vi "Initialize.vi"(7 "Serial Configuration":T1={"Baud Rate"=9600, "Parity"=1, "Data Bits"=7, "Stop Bits"=10, "Flow Control"=0} {"Flow Control" items=["None", "XON/XOFF", "RTS/CTS", "XON/XOFF & RTS/CTS", "DTR/DSR", "XON/XOFF & DTR/DSR"]; "Stop Bits" items=["1.0"=10, "1.5"=15, "2.0"=20]; "Data Bits" items=["7"=7, "8"=8]; "Parity" items=["None", "Odd", "Even", "Mark", "Space"]; "Baud Rate" items=["300"=300, "600"=600, "1200"=1200, "2400"=2400, "4800"=4800, "9600"=9600, "19200"=19200, "38400"=38400, "57600"=57600]}, 8 "error in (no error)":errorcluster, 9 "Reset (True)":bool=TRUE, 10 "ID Query (True)":bool=TRUE, 11 "VISA resource name":refnum<visa-resource-name>="GPIB0::12::INSTR") -> (0 "error out":errorcluster, 3 "VISA resource name out":refnum<visa-resource-name>)   [LabVIEW 2019, in "Lake Shore 325.lvlib"]
doc: "Establishes communication with the instrument and optionally performs an instrument identification query and/or an instrument reset. It also places the instrument in a default state needed for other instrument driver operations. Therefore, call this VI before calling other instrument driver VIs for this instrument. Generally, you need to call the <B>Initialize VI</B> only once at the beginning of an application."
uses:
  <instrlib>/Lake Shore 325/Lake Shore 325.lvlib
panel:
  # "© 2006 Lake Shore Cryotronics Inc.  ALL RIGHTS RESERVED."
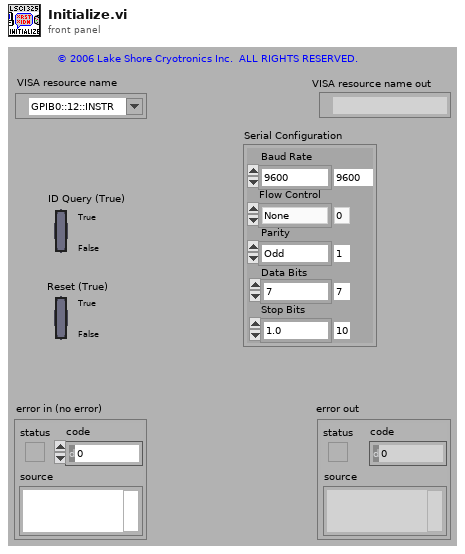
[diagram p1: front panel]
types:
  T1 = cluster{"Baud Rate":u32, "Parity":u16, "Data Bits":u16, "Stop Bits":u16, "Flow Control":u16}
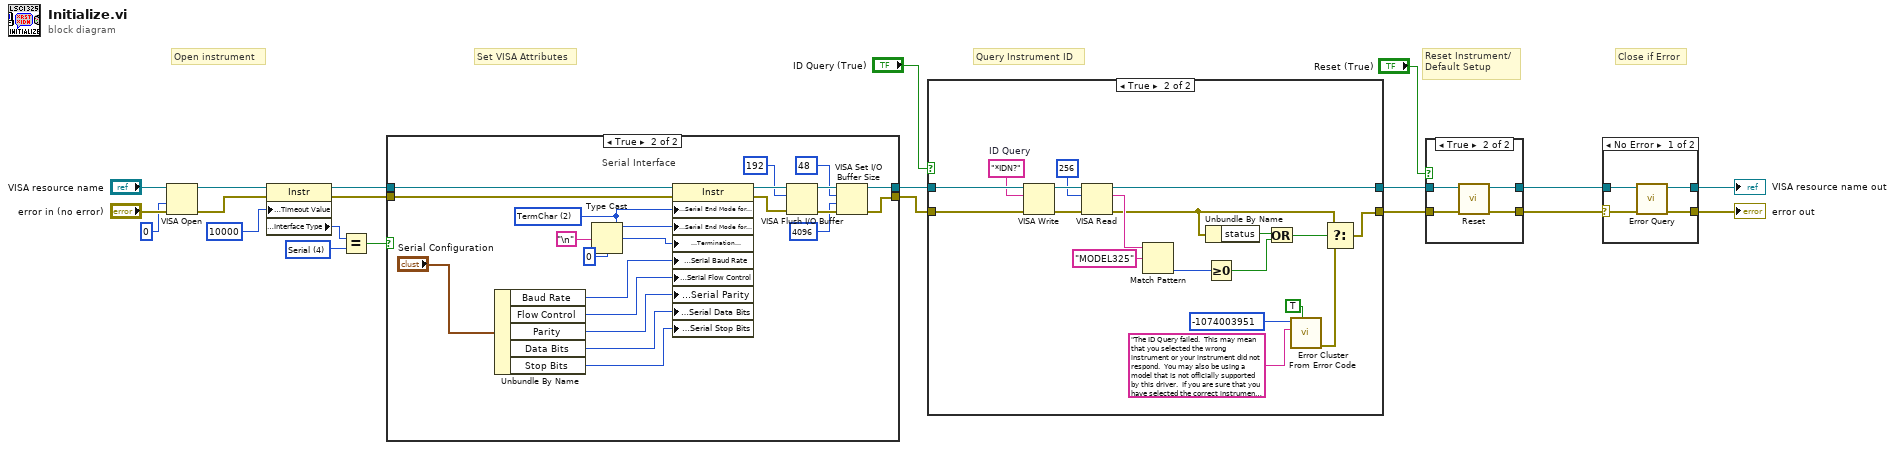
[diagram p0: block diagram]
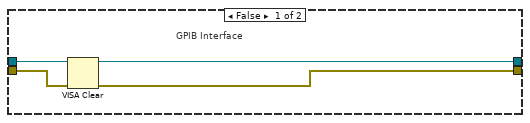
[diagram p2: hidden frame]
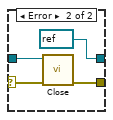
[diagram p3: hidden frame]
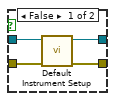
[diagram p4: hidden frame]
diagram:
  w8 = u16 4 items=["GPIB"=1, "VXI"=2, "GPIB-VXI"=3, "Serial"=4, "PXI"=5, "TCPIP"=6, "USB"=7] ("Interface Information:Interface Type")
  # "Set VISA Attributes"
  # "Close if Error"
  # "Query Instrument ID"
  # "Reset Instrument/\nDefault Setup"
  # "Open instrument"
  n1 = VISA Open(access mode=u32 0, error in (no error)="error in (no error)", VISA resource name="VISA resource name") -> (VISA resource name=w2:refnum<visa-resource-name>, error out=w1:errorcluster)  [unwired: 2 in]
  n2 = property class="Instr"(reference=w2, error in=w1, "General Settings:Timeout Value"=u32 10000) -> (reference out=w11:refnum<visa-resource-name>, error out=w10:errorcluster, "Interface Information:Interface Type"=w15:u16)
  n3 = Equal?(x=w15, y=w8) -> (x = y?=w9:bool)
  n4 = case shown="True" w9 {
    tunnel: [w23 w43] -> w13
    tunnel: [w22 w40] -> w12
    tunnel: w11 -> [w25 w45]
    tunnel: w10 -> [w24 w46]
    frame False {
      # "GPIB Interface"
      n5 = VISA Clear(VISA resource name=w25, error in (no error)=w24) -> (VISA resource name out=w23:refnum<visa-resource-name>, error out=w22:errorcluster)
    }
    frame True {
      w34 = u16 2 items=["None", "LastBit", "TermChar"] ("Serial Settings:Serial End Mode for Reads")
      # "Serial Interface"
      n6 = Unbundle By Name("Serial Configuration") -> ("Baud Rate"=w32:u32, "Flow Control"=w28:u16, "Parity"=w30:u16, "Data Bits"=w31:u16, "Stop Bits"=w27:u16)
      n7 = Type Cast(type=u8 0, x="\n") -> (*(type *) &x=w33:u8)
      n8 = property class="Instr"(reference=w45, error in=w46, "Serial Settings:Serial End Mode for Reads"=w34, "Serial Settings:Serial End Mode for Writes"=w34, "Message Based Settings:Termination Character"=w33, "Serial Settings:Serial Baud Rate"=w32, "Serial Settings:Serial Flow Control"=w28, "Serial Settings:Serial Parity"=w30, "Serial Settings:Serial Data Bits"=w31, "Serial Settings:Serial Stop Bits"=w27) -> (reference out=w39:refnum<visa-resource-name>, error out=w42:errorcluster)
      n9 = VISA Flush I/O Buffer(VISA resource name=w39, mask (16)=u16 192, error in (no error)=w42) -> (VISA resource name out=w44:refnum<visa-resource-name>, error out=w41:errorcluster)
      n10 = VISA Set I/O Buffer Size(VISA resource name=w44, mask (16)=u16 48, size (4096)=u32 4096 ("size (0)"), error in (no error)=w41) -> (VISA resource name out=w43:refnum<visa-resource-name>, error out=w40:errorcluster)
    }
  }
  n11 = case shown="True" "ID Query (True)" {
    tunnel: [w47 w67] -> w20
    tunnel: [w48 w50] -> w21
    tunnel: w13 -> [w48 w65]
    tunnel: w12 -> [w47 w66]
    frame False {
    }
    frame True {
      w51 = "*IDN?"  # ID Query
      n12 = VISA Write(VISA resource name=w65, write buffer=w51, error in (no error)=w66) -> (VISA resource name out=w63:refnum<visa-resource-name>, error out=w62:errorcluster)  [unwired: 1 out]
      n13 = VISA Read(VISA resource name=w63, byte count=u32 256, error in (no error)=w62) -> (VISA resource name out=w50:refnum<visa-resource-name>, read buffer=w64:string, error out=w49:errorcluster)  [unwired: 1 out]
      n14 = Match Pattern(string=w64, regular expression="MODEL325") -> (offset past match=w55:i32)  [unwired: 1 in, 3 out]
      n15 = Unbundle By Name(w49) -> ("status"=w54:bool)
      n16 = Greater Or Equal To 0?(x=w55) -> (x >= 0?=w52:bool)
      n17 = Or(x=w54, y=w52) -> (x .or. y?=w53:bool)
      n18 = call <vilib>:"Error Cluster From Error Code.vi"("show call chain? (False)"=TRUE, "error message (\"\")"="The ID Query failed.  This may mean that you selected the wrong instrument or your instrument did not respond.  You may also be using a model that is not officially supported by this driver.  If you are sure that you have selected the correct instrument and it is responding, try disabling the ID Query." ("Source (VI Name)"), "error code (0)"=-1074003951 ("Code")) -> ("error out"=w59:errorcluster)  [unwired: 6 in]
      n19 = Select(t=w49, s=w53, f=w59) -> (s? t:f=w67:errorcluster)
    }
  }
  n20 = case shown="True" "Reset (True)" {
    tunnel: w20 -> [w70 w72]
    tunnel: [w69 w75] -> w3
    tunnel: w21 -> [w71 w73]
    tunnel: [w68 w74] -> w4
    frame False {
      n21 = call <instrlib>:"Default Instrument Setup.vi"("error in (no error)"=w70, "VISA resource name"=w71) -> ("error out"=w69:errorcluster, "VISA resource name out"=w68:refnum<visa-resource-name>)  [unwired: 8 in]
    }
    frame True {
      n22 = call <instrlib>:"Reset.vi"("error in (no error)"=w72, "VISA resource name"=w73) -> ("error out"=w75:errorcluster, "VISA resource name out"=w74:refnum<visa-resource-name>)  [unwired: 8 in]
    }
  }
  n23 = case shown="No Error" w3 {
    selector: w3 -> [w79 w81]
    tunnel: w4 -> [w78 w82]
    tunnel: [w77 refnum<visa-resource-name> refnum ("VISA resource name out")] -> w6
    tunnel: [w76 w83] -> w5
    frame No Error {
      n24 = call <instrlib>:"Error Query.vi"("error in (no error)"=w79, "VISA resource name"=w78) -> ("error out"=w76:errorcluster, "VISA resource name out"=w77:refnum<visa-resource-name>)  [unwired: 7 in, 1 out]
    }
    frame Error {
      n25 = call <instrlib>:"Close.vi"("error in (no error)"=w81, "VISA resource name"=w82) -> ("error out"=w83:errorcluster)  [unwired: 9 in]
    }
  }
  "VISA resource name out" <- w6
  "error out" <- w5
